vi "getAnalysisPath.vi"(8 "error in (no error)":errorcluster, 11 "FileNeologist in":refnum<class "FileNeologist.lvclass">) -> (0 "error out":errorcluster, 2 "AbsorptionAnalysisPath":path, 3 "FileNeologist out":refnum<class "FileNeologist.lvclass">)   [LabVIEW 2011, in "Tools.lvlib" / "Filing.lvlib" / "FileNeologist.lvclass"]
uses:
  FileNeologist.lvclass
  FileNeologist.lvclass/FileNeologist.ctl
  FileSystem/FileSystem.lvclass
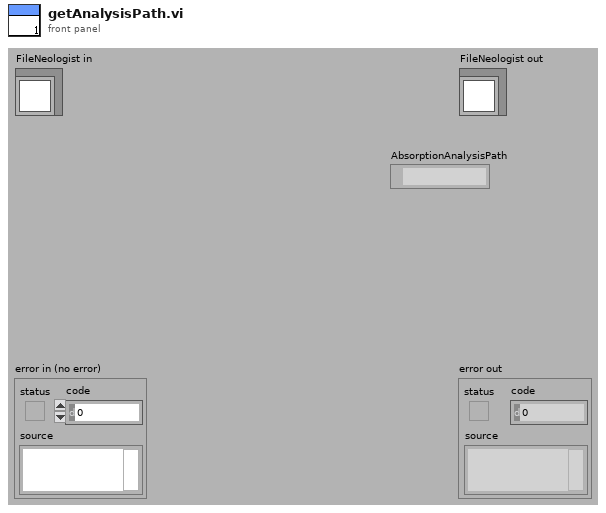
[diagram p1: front panel]
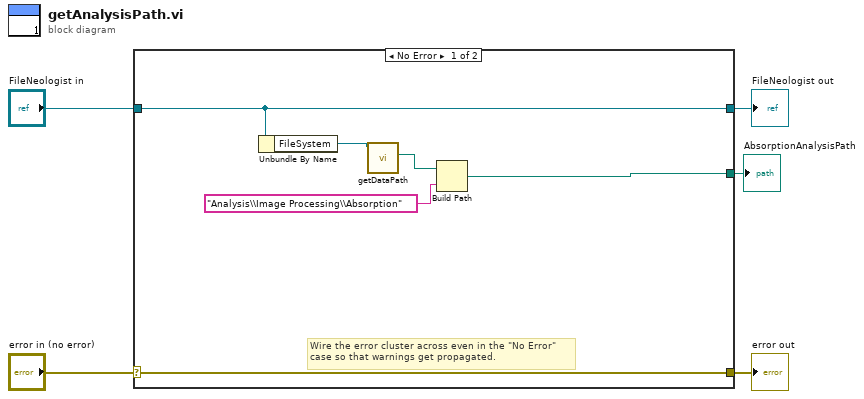
[diagram p0: block diagram]
diagram:
  n1 = case shown="No Error" "error in (no error)" {
    selector: "error in (no error)" -> [w11 w13]
    tunnel: [w11 w13] -> w4
    tunnel: [w10 w12] -> w2
    tunnel: "FileNeologist in" -> [w10 w12]
    tunnel: [w6 _] -> w1
    frame No Error {
      # "Wire the error cluster across even in the \"No Error\"\ncase so that warnings get propagated."
      n2 = Unbundle By Name(w10) -> ("FileSystem"=w9:refnum<class "FileSystem.lvclass">)
      n3 = call-dynamic "getDataPath.vi"("FileSystem.lvclass in"=w9) -> ("DataPath"=w8:path)  [unwired: 8 in, 2 out]
      n4 = Build Path(base path=w8, name or relative path="Analysis\\Image Processing\\Absorption") -> (appended path=w6:path)
    }
    frame Error {
    }
  }
  "error out" <- w4
  "FileNeologist out" <- w2
  "AbsorptionAnalysisPath" <- w1
